vi "Keithley 24XX Read Multiple.vi"() -> ()   [LabVIEW 2019]
doc: "This example shows how to configure a measurement and take multiple readings."
uses:
  Public/Data/Read (Multiple Points).vi
  Keithley 24XX.lvlib
panel:
  in  "Source Mode  (0: Voltage)":u16(ring) items=["Voltage", "Current"]
  in  "Output Level (0)":dbl
  in  "Compliance  Level (0.1)":dbl=0.1
  in  "Timeout (10000 ms)":i32=10000 format="%#.6g"
  in  "Sample Count (10)":i32=10
  out "Resistance":sgl[](array[numeric])
  out "Current":sgl[](array[numeric])
  out "Voltage":sgl[](array[numeric])
  in  "Serial Configuration":T1={"Baud Rate"=9600, "Parity"=0, "Data Bits"=8, "Stop Bits"=10, "Flow Control"=0} {"Flow Control" items=["None", "XON/XOFF", "RTS/CTS", "XON/XOFF & RTS/CTS", "DTR/DSR", "XON/XOFF & DTR/DSR"]; "Stop Bits" items=["1.0"=10, "1.5"=15, "2.0"=20]; "Data Bits" items=["7"=7, "8"=8]; "Parity" items=["None", "Odd", "Even", "Mark", "Space"]; "Baud Rate" items=["300"=300, "600"=600, "1200"=1200, "2400"=2400, "4800"=4800, "9600"=9600, "19200"=19200]}
  in  "VISA resource name":refnum<visa-resource-name>
  # "(c) 2006 - 2015 National Instruments.  ALL RIGHTS RESERVED."
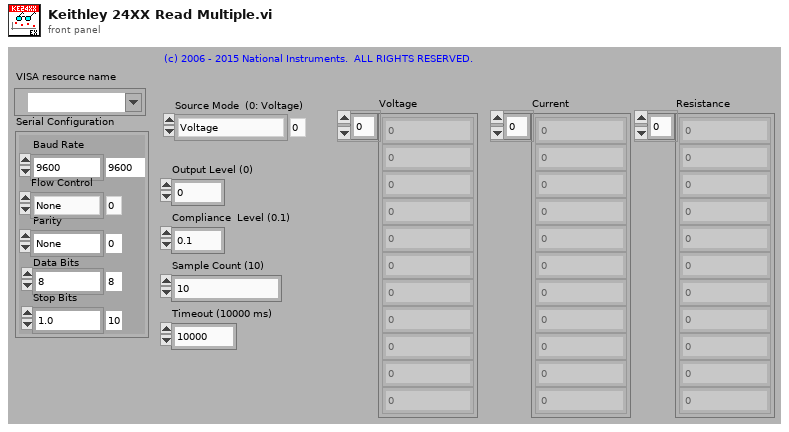
[diagram p1: front panel]
types:
  T1 = cluster{"Baud Rate":u32, "Parity":u16, "Data Bits":u16, "Stop Bits":u16, "Flow Control":u16}
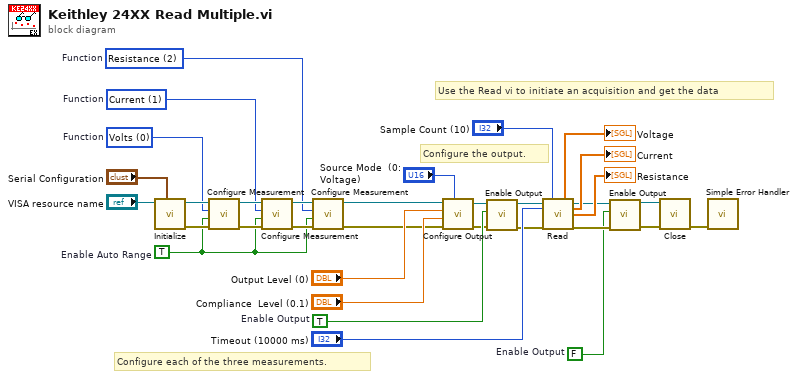
[diagram p0: block diagram]
diagram:
  w8 = TRUE  # Enable Output
  w9 = FALSE  # Enable Output
  w21 = u16 2 items=["Volts", "Current", "Resistance"]  # Function
  w22 = u16 1 items=["Volts", "Current", "Resistance"]  # Function
  w23 = u16 0 items=["Volts", "Current", "Resistance"]  # Function
  w24 = TRUE  # Enable Auto Range
  # "Use the Read vi to initiate an acquisition and get the data"
  # "Configure the output."
  # "Configure each of the three measurements."
  n1 = call "Initialize.vi"("Serial Configuration"="Serial Configuration", "VISA resource name"="VISA resource name") -> ("error out"=w30:errorcluster, "VISA resource name out"=w31:refnum<visa-resource-name>)  [unwired: 8 in]
  n2 = call "Configure Measurement.vi"("error in (no error)"=w30, "Enable Auto Range (T:Enable)"=w24, "Function (0: Volts)"=w23, "VISA resource name"=w31) -> ("error out"=w28:errorcluster, "VISA resource name out"=w27:refnum<visa-resource-name>)  [unwired: 6 in]
  n3 = call "Configure Measurement.vi"("error in (no error)"=w28, "Enable Auto Range (T:Enable)"=w24, "Function (0: Volts)"=w22, "VISA resource name"=w27) -> ("error out"=w25:errorcluster, "VISA resource name out"=w26:refnum<visa-resource-name>)  [unwired: 6 in]
  n4 = call "Configure Measurement.vi"("error in (no error)"=w25, "Enable Auto Range (T:Enable)"=w24, "Function (0: Volts)"=w21, "VISA resource name"=w26) -> ("error out"=w6:errorcluster, "VISA resource name out"=w7:refnum<visa-resource-name>)  [unwired: 6 in]
  n5 = call "Configure Output.vi"("Source Mode  (0: Voltage)"="Source Mode  (0: Voltage)", "error in (no error)"=w6, "Compliance  Level (0.1)"="Compliance  Level (0.1)", "Output Level (0)"="Output Level (0)", "VISA resource name"=w7) -> ("error out"=w2:errorcluster, "VISA resource name out"=w3:refnum<visa-resource-name>)  [unwired: 5 in]
  n6 = call "Enable Output.vi"("error in (no error)"=w2, "Enable Output (T: Enable)"=w8, "VISA resource name"=w3) -> ("error out"=w5:errorcluster, "VISA resource name out"=w4:refnum<visa-resource-name>)  [unwired: 7 in]
  n7 = call-poly "Read.vi"("VISA resource name"=w4, "Sample Count (1)"="Sample Count (10)", "Timeout (10000 ms)"="Timeout (10000 ms)", "error in (no error)"=w5) -> ("Voltage"=→"Voltage":sgl[], "VISA resource name out"=w11:refnum<visa-resource-name>, "Current"=→"Current":sgl[], "Resistance"=→"Resistance":sgl[], "error out"=w10:errorcluster)  [unwired: 5 in, 2 out]
  n8 = call "Enable Output.vi"("error in (no error)"=w10, "Enable Output (T: Enable)"=w9, "VISA resource name"=w11) -> ("error out"=w12:errorcluster, "VISA resource name out"=w13:refnum<visa-resource-name>)  [unwired: 7 in]
  n9 = call "Close.vi"("error in (no error)"=w12, "VISA resource name"=w13) -> ("error out"=w33:errorcluster)  [unwired: 9 in]
  n10 = call <vilib>:"Simple Error Handler.vi"("error in (no error)"=w33) -> ()  [unwired: 4 in, 5 out]
